vi "ManualTestingDialog.vi"(8 "error in":errorcluster) -> (0 "error out":errorcluster, 1 "检测区域":string, 2 "是否采样":bool, 3 "采样信息":T1, 4 "电压倍数":string, 5 "设置电源电压05V":string)   [LabVIEW 2014, in "Sample.lvlib"]
uses:
  Sample.lvlib
  DataBase/DataBase.lvlib
  DetectElecrodes/DetectElectros.lvlib
panel:
  out "电压范围":string
  out "电压频率":string
  out "输出电压值":string
  in  "备注":string
  in  "退出按钮":bool
  in  "开始采样":bool
  in  "电源电流":string
  in  "电源电压":string
  in  "电源频率":string="1"
  in  "采样位置":u16(ring) items=["上层膜采样", "下层膜采样"]
  in  "OK":bool
  in  "检测区域":u16(ring) items=["1区", "2区"]
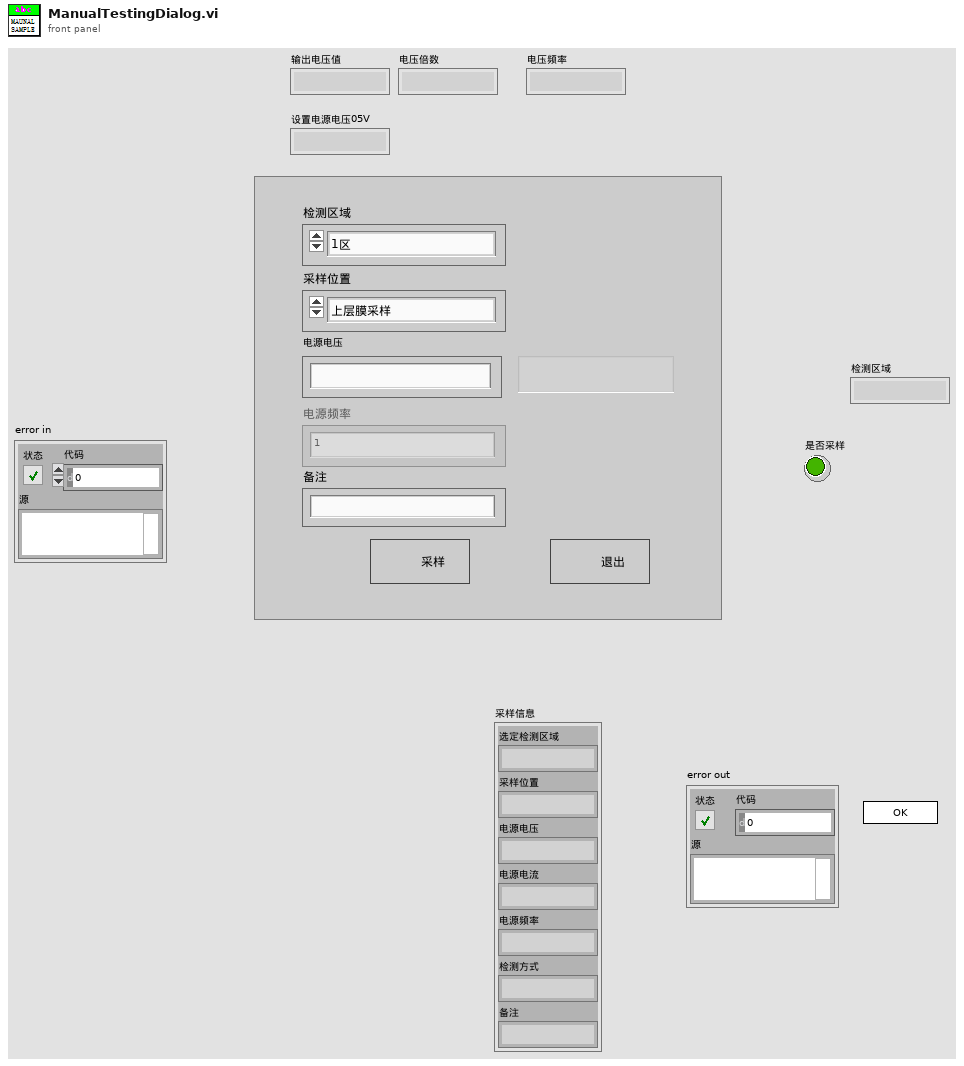
[diagram p1: front panel]
types:
  T1 = cluster{"选定检测区域":string, "采样位置":string, "电源电压":string, "电源电流":string, "电源频率":string, "检测方式":string, "备注":string}
  T2 = enum32{"invalid app kind", "Development System", "Run Time System", "Student Edition", "Embedded LabVIEW", "Evaluation", "Custom"}
  T3 = enum32{"Invalid", "Standard", "Closed", "Hidden", "Minimized", "Maximized"}
  T4 = cluster{"Core":cluster{"Current VI Reference":refnum<vi>, "Close Panel on Exit?":bool}, "Your Boolean data":bool, "Your string data":string, "采样位置":string, "检测区域":string[], "选定检测区域":cluster{"选定检测区域":string, "序号":i32}, "输出电压值":string, "电压频率":string, "电压倍数":string, "采样信息":cluster{"选定检测区域":string, "采样位置":string, "电源电压":string, "电源电流":string, "电源频率":string, "检测方式":string, "备注":string}, "最大电压":i32}
  T5 = cluster{"Current VI Reference":refnum<vi>, "Close Panel on Exit?":bool}
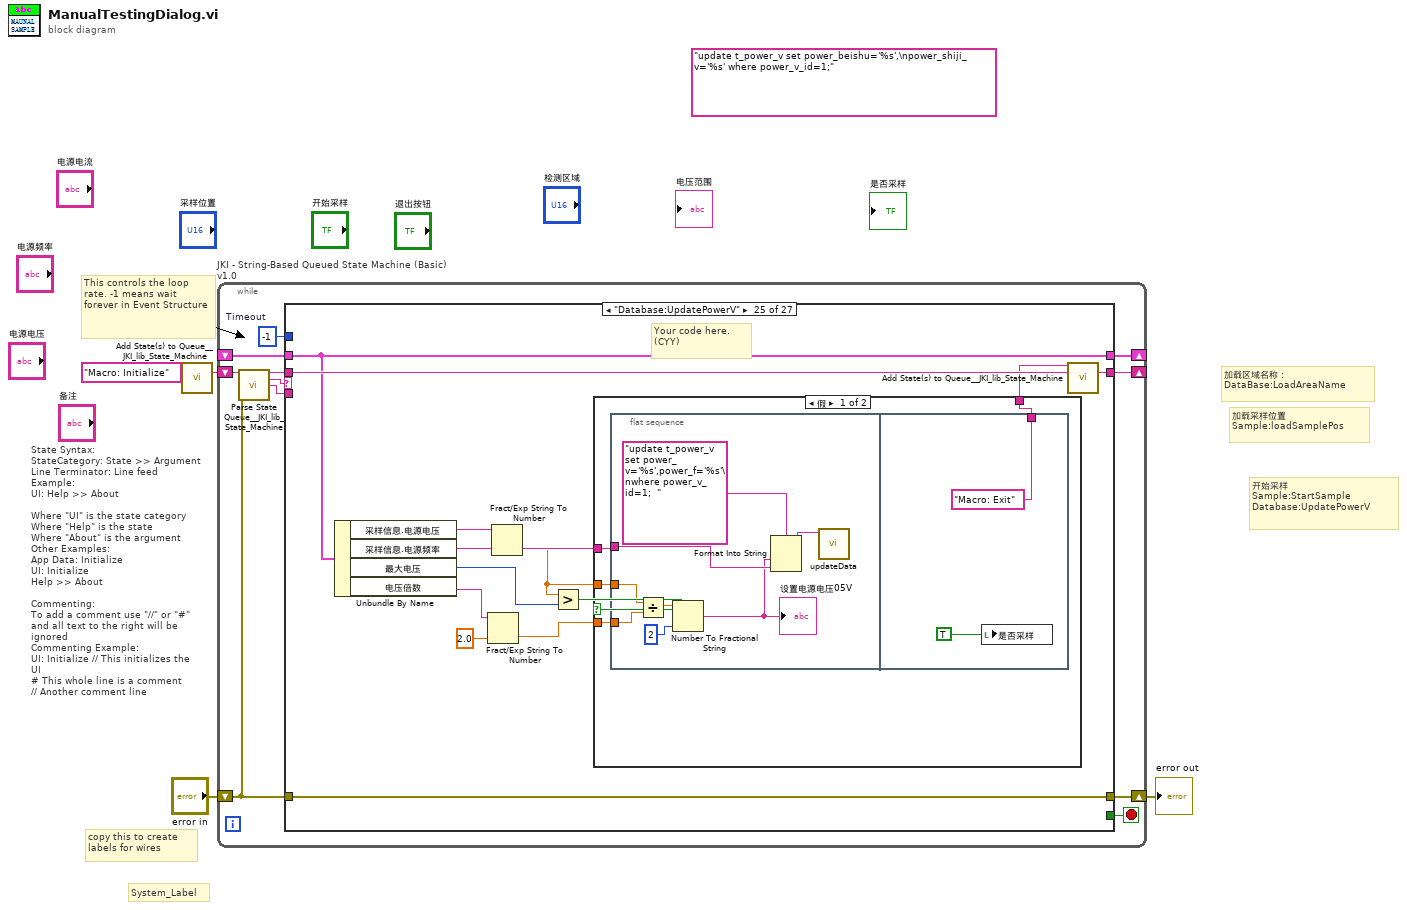
[diagram p0: block diagram]
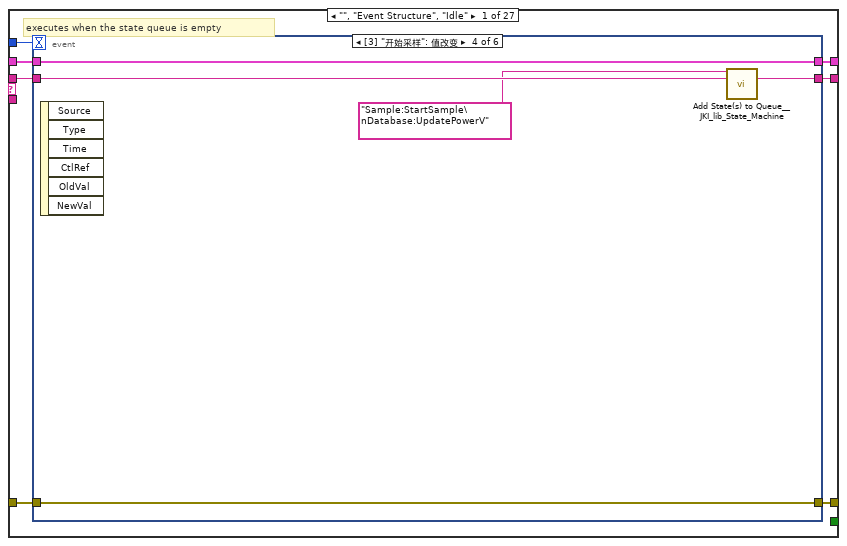
[diagram p2: hidden frame]
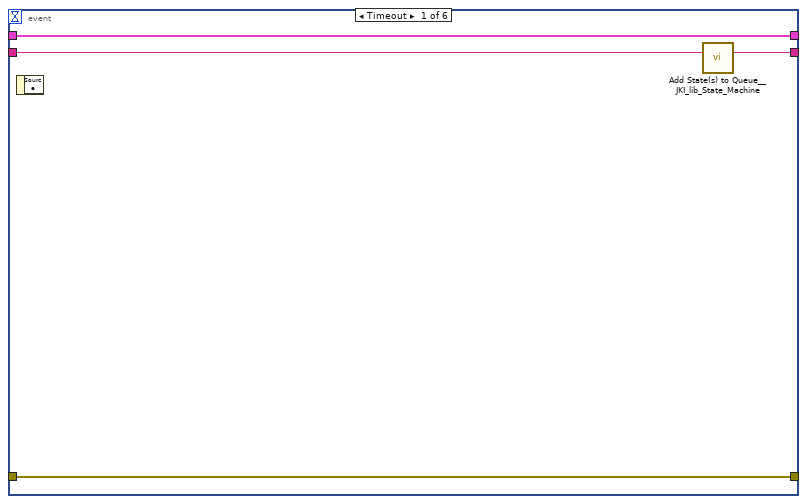
[diagram p3: hidden frame]
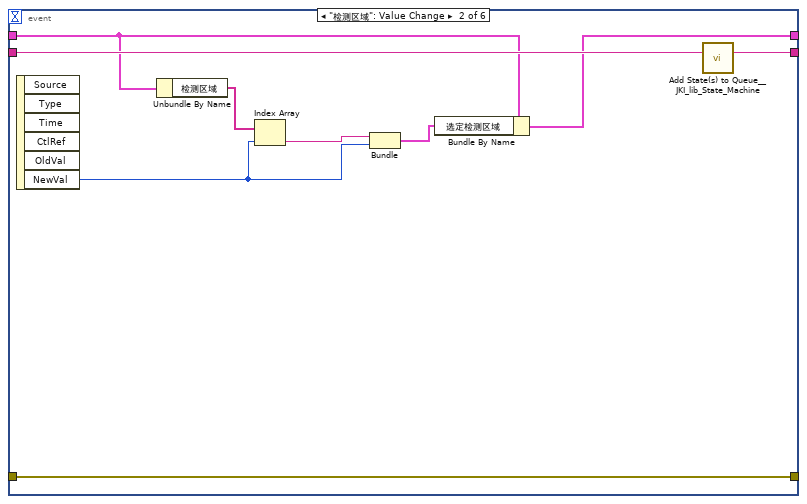
[diagram p4: hidden frame]
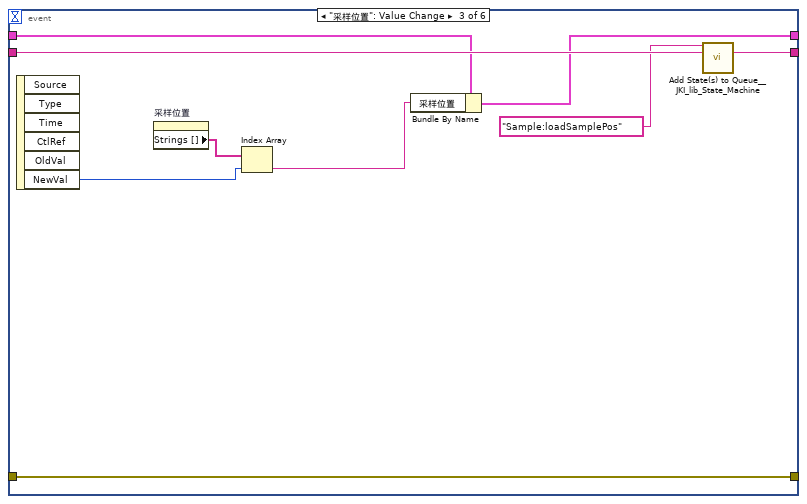
[diagram p5: hidden frame]
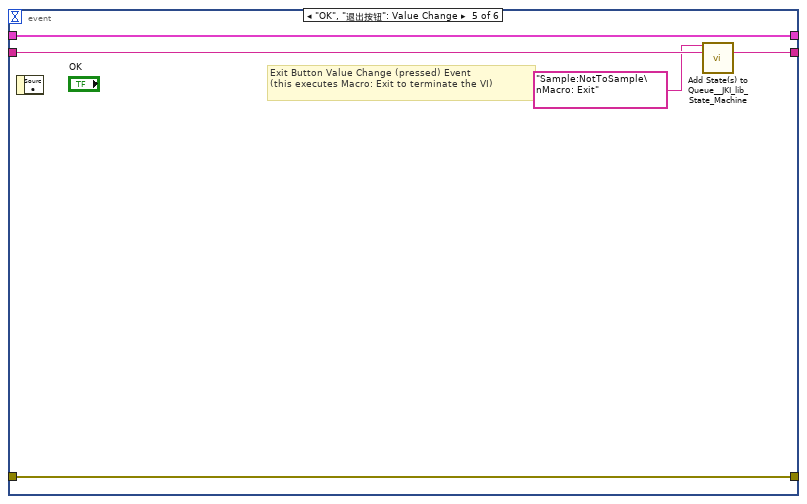
[diagram p6: hidden frame]
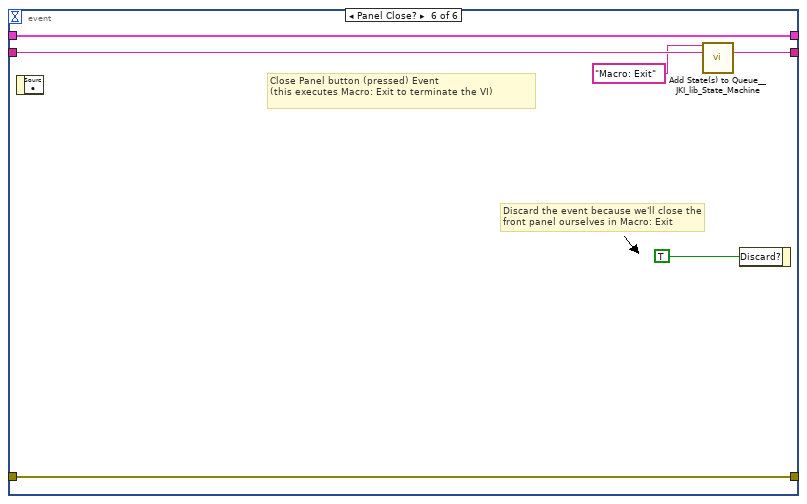
[diagram p7: hidden frame]
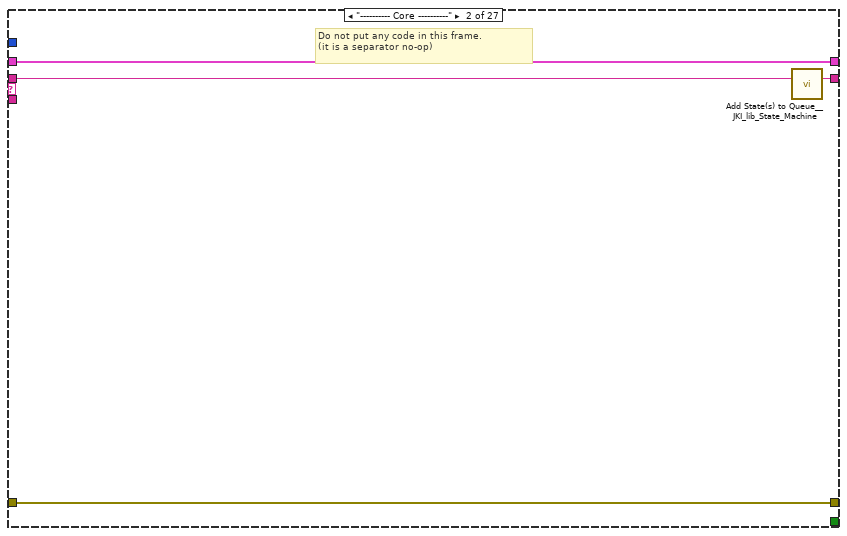
[diagram p8: hidden frame]
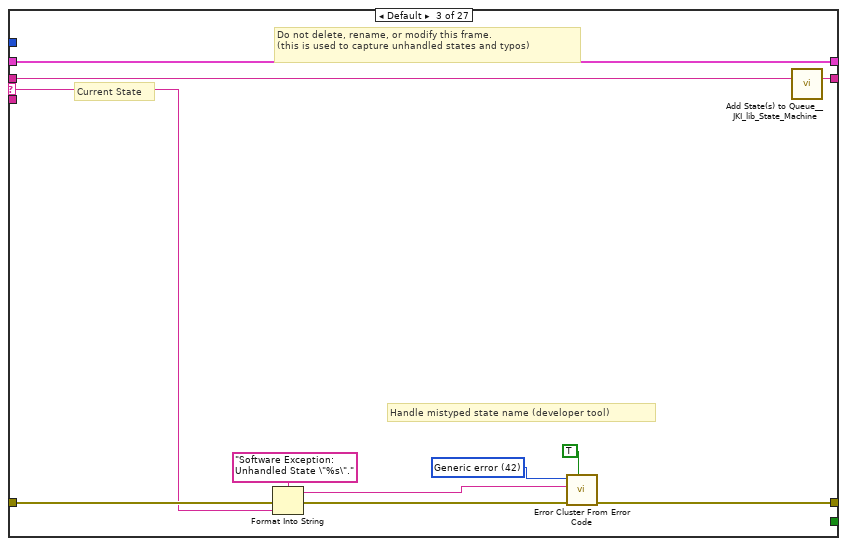
[diagram p9: hidden frame]
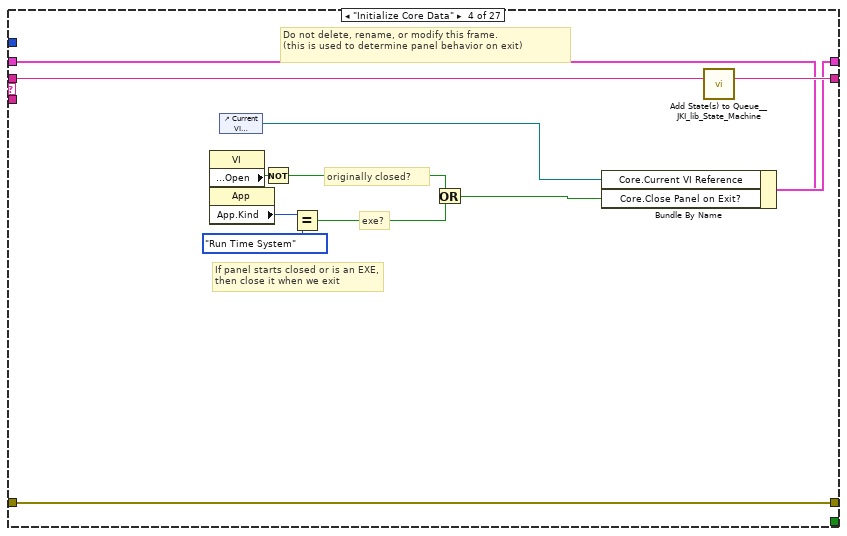
[diagram p10: hidden frame]
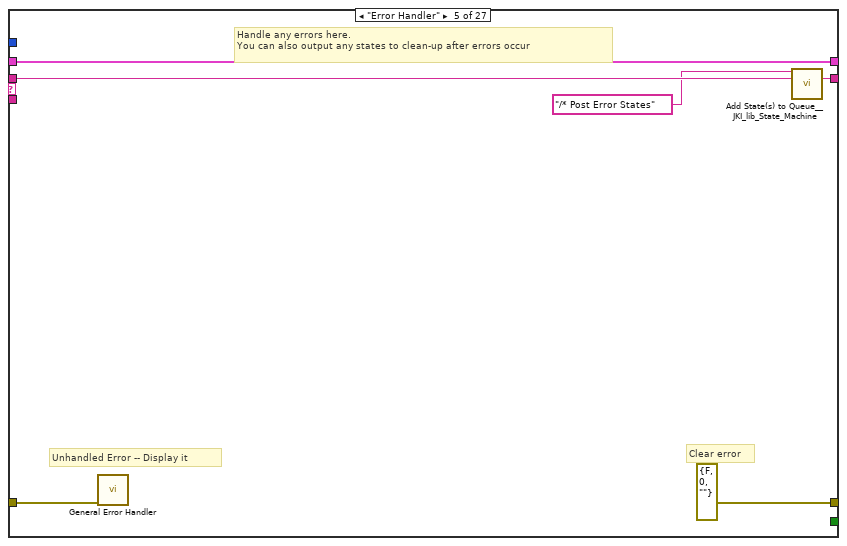
[diagram p11: hidden frame]
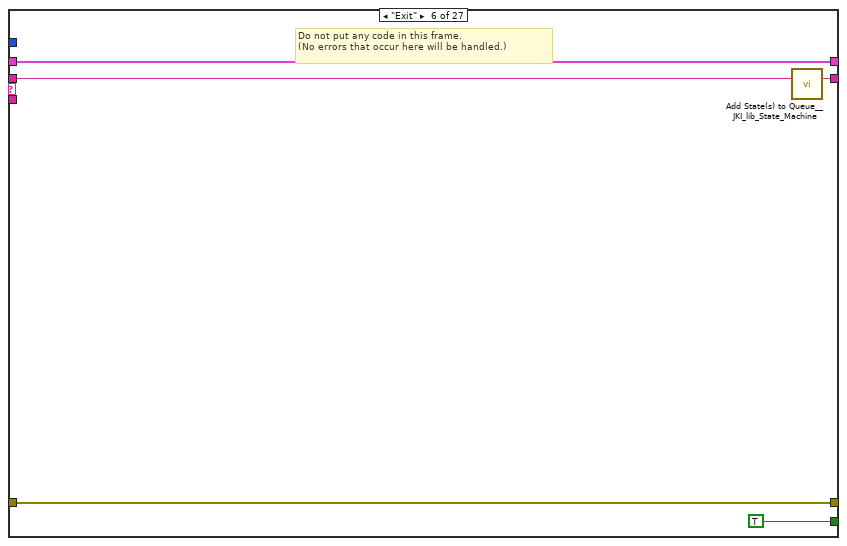
[diagram p12: hidden frame]
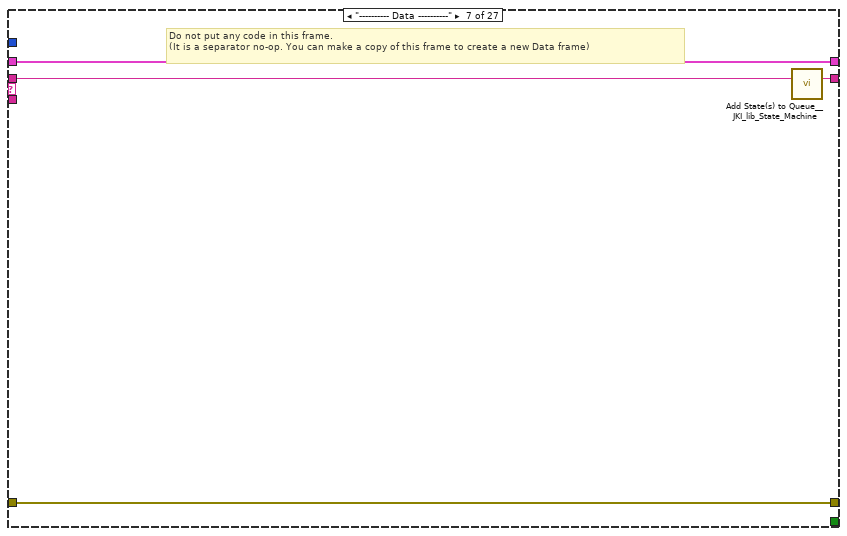
[diagram p13: hidden frame]
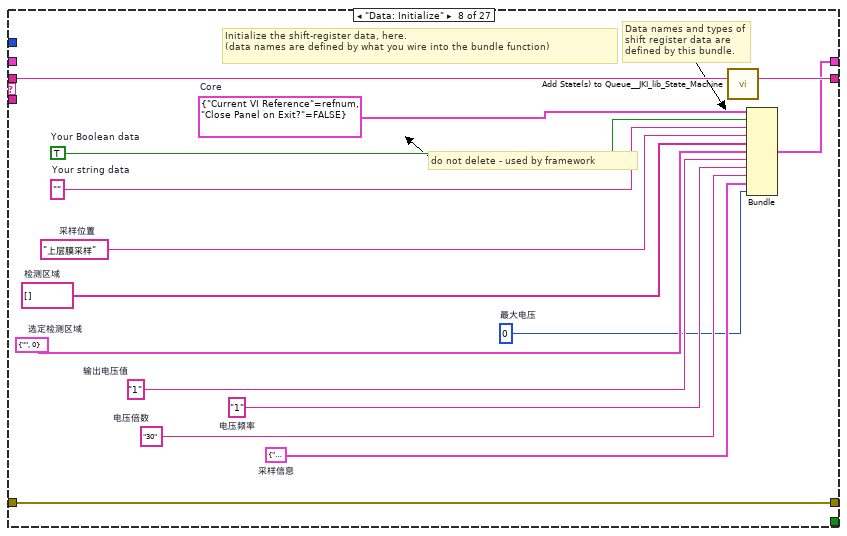
[diagram p14: hidden frame]
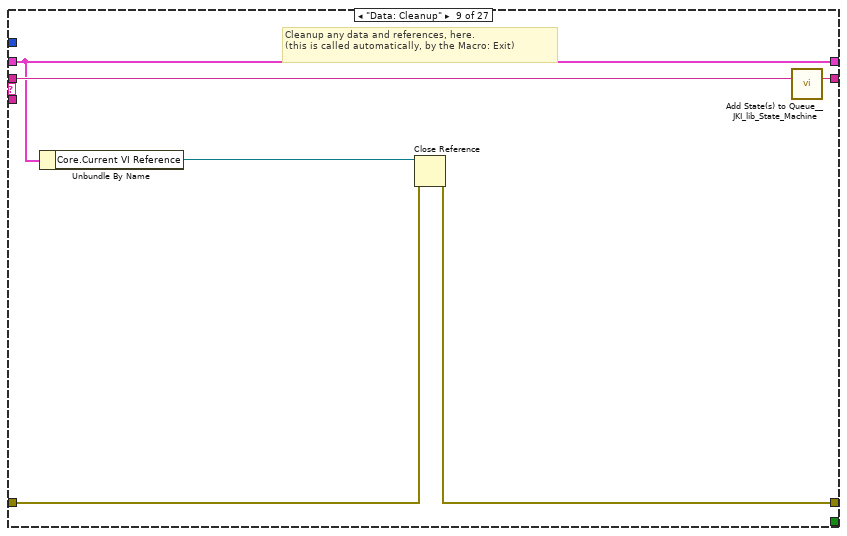
[diagram p15: hidden frame]
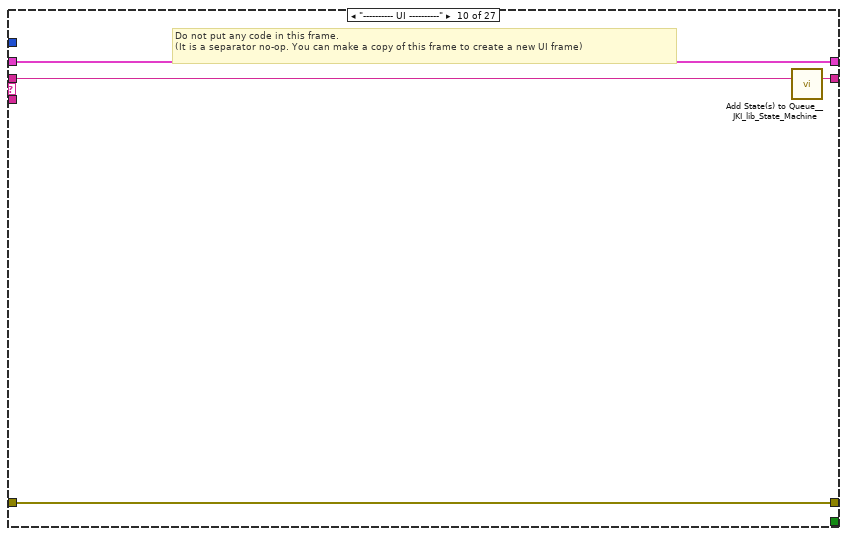
[diagram p16: hidden frame]
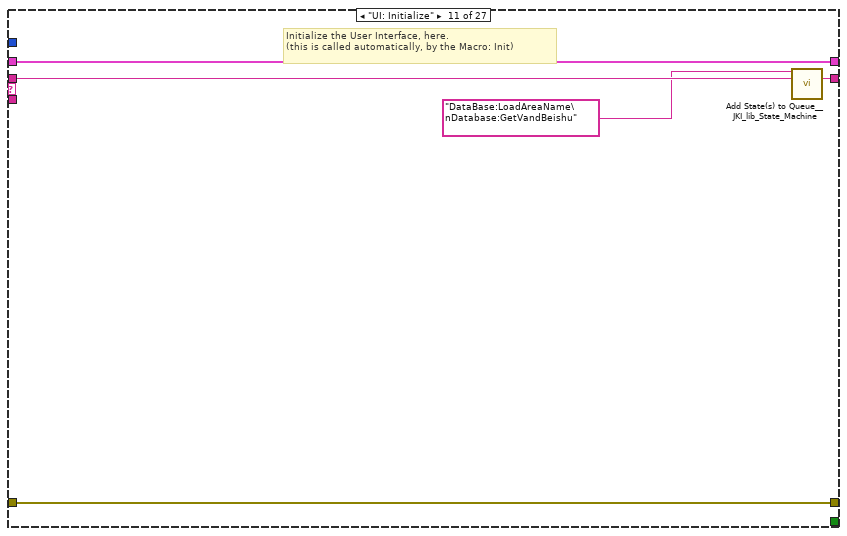
[diagram p17: hidden frame]
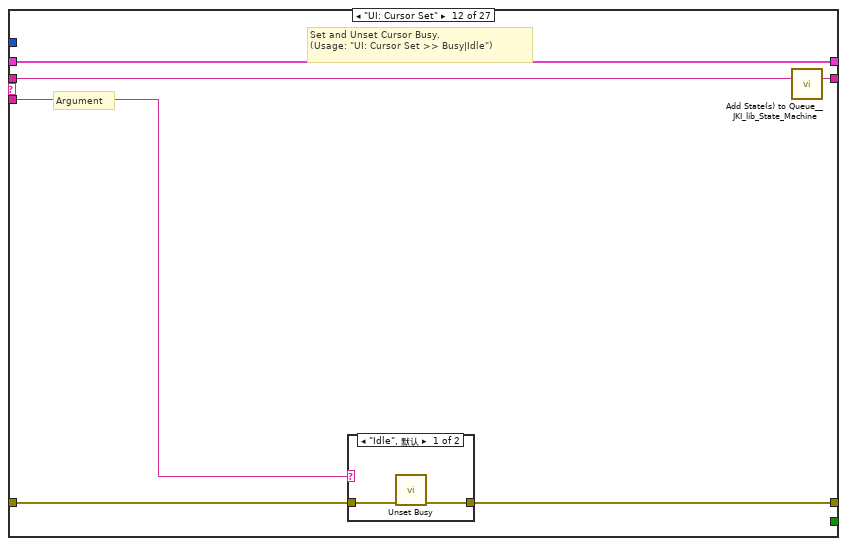
[diagram p18: hidden frame]
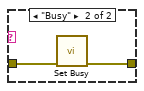
[diagram p19: hidden frame]
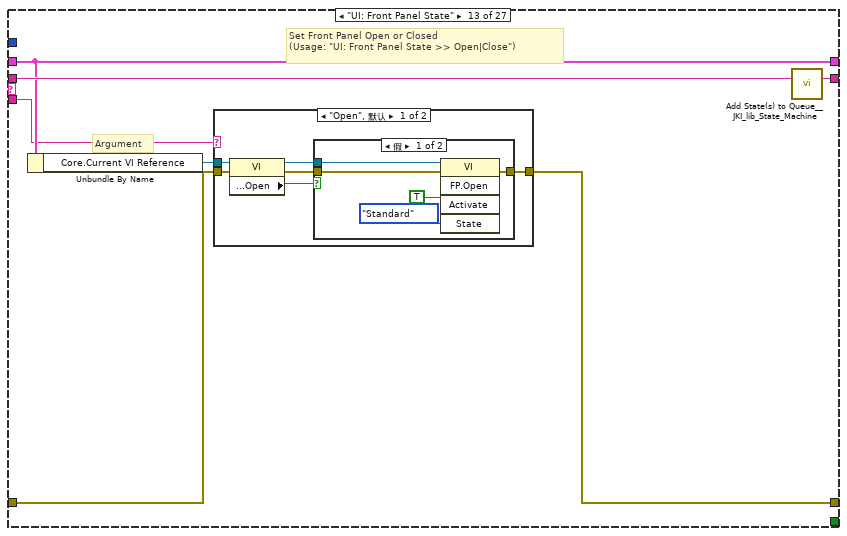
[diagram p20: hidden frame]
diagram:
  (unwired) "update t_power_v set power_beishu='%s',\npower_shiji_v='%s' where power_v_id=1;"
  # "开始采样\nSample:StartSample\nDatabase:UpdatePowerV"
  # "加载采样位置\nSample:loadSamplePos"
  # "加载区域名称：\nDataBase:LoadAreaName"
  # "State Syntax:\nStateCategory: State >> Argument\nLine Terminator: Line feed\nExample:\nUI: Help >> About\n\nWhere \"UI\" is the state category\nWhere \"Help\" is the state\nWhere \"About\" is the argument\nOther Examples:\nApp Data: Initialize\nUI: Initialize\nHelp >> About\n\nCommenting:\nTo add a comment use \"//\" or \"#\" and all text to the right will be ignored\nCommenting Example:\nUI: Initialize // This initializes the UI\n# This whole line is a comment\n// Another comment line"
  # "copy this to create labels for wires"
  # "This controls the loop rate. -1 means wait forever in Event Structure"
  # "System_Label"
  n1 = call <vilib>:"Add State(s) to Queue__JKI_lib_State_Machine.vi"("State(s) in (\"\")"="Macro: Initialize") -> ("States Out"=w4:string)  [unwired: 14 in]
  n2 = while "JKI - String-Based Queued State Machine (Basic) v1.0" {
    shift-right: [w8] -> _
    shift-left: _ -> [w7]
    shift-right: [w11] -> w2
    shift-left: "error in" -> [w5]
    shift-right: [w10] -> _
    shift-left: w4 -> [w12]
    stop <- w9 stop-if-true
    w6 = -1  # Timeout
    n3 = call <vilib>:"Parse State Queue__JKI_lib_State_Machine.vi"("State Queue"=w12, "Error In (no error)"=w5) -> ("Remaining States"=w14:string, "Current State"=w15:string, "Arguments"=w13:string)  [unwired: 11 in]
    n4 = case shown="\"Database:UpdatePowerV\"" w15 {
      selector: w15 -> [_ _ w65 _ _ _ _ _ _ _ _ _ _ _ _ _ _ _ _ _ _ _ _ _ _ _ _]
      tunnel: w14 -> [w22 w64 w69 w87 w93 w98 w102 w117 w123 w127 w132 w138 w149 w175 w180 w190 w194 w198 w202 w206 w211 w229 w233 w237 w250 w277 w291]
      tunnel: w13 -> [_ _ _ _ _ _ _ _ _ _ _ w133 w143 _ _ _ _ _ _ _ _ _ _ _ _ _ _]
      tunnel: w7 -> [w20 w61 w67 w78 w90 w96 w99 _ w118 w124 w130 w136 w145 w172 w177 w187 w191 w195 w199 w203 w208 w213 w230 w234 w247 w272 w282]
      tunnel: [w19 w62 w71 w84 errorcluster {"status"=FALSE, "code"=0, "source"=""} ("error out") w95 w100 w114 w119 w125 w129 w134 w146 w173 w178 w188 w192 w196 w200 w204 w209 w227 w231 w235 w248 w275 w289] -> w11
      tunnel: w5 -> [w18 w62 w70 w84 w89 w95 w100 w114 w120 w125 w129 w135 w147 w173 w178 w188 w192 w196 w200 w204 w209 w227 w231 w235 w248 w275 w289]
      tunnel: [w21 w63 w68 w86 w92 w97 w101 w116 w122 w126 w131 w137 w148 w174 w179 w189 w193 w197 w201 w205 w210 w228 w232 w236 w249 w276 w290] -> w10
      tunnel: [_ _ _ _ _ TRUE _ _ _ _ _ _ _ _ _ _ _ _ _ _ _ _ _ _ _ _ _] -> w9
      tunnel: [w17 w61 w67 w85 w90 w96 w99 w115 w118 w124 w130 w136 w145 w172 w177 w187 w191 w195 w199 w203 w208 w212 w230 w234 w247 w271 w281] -> w8
      tunnel: w6 -> [w16 _ _ _ _ _ _ _ _ _ _ _ _ _ _ _ _ _ _ _ _ _ _ _ _ _ _]
      frame "", "Event Structure", "Idle" {
        # "executes when the state queue is empty"
        n5 = event shown="[3] \"开始采样\": 值改变" {
          selector: _ -> [_ _ _ _ _ _]
          dyn-events: _ -> [_ _ _ _ _ _]
          timeout: w16 -> [_ _ _ _ _ _]
          tunnel: w22 -> [w26 w35 w44 w49 w54 w60]
          tunnel: [w25 w34 w43 w48 w53 w59] -> w21
          tunnel: w20 -> [w23 w31 w38 w46 w51 w57]
          tunnel: [w24 w33 w42 w47 w52 w58] -> w19
          tunnel: w18 -> [w24 w33 w42 w47 w52 w58]
          tunnel: [w23 w30 w37 w46 w51 w57] -> w17
          event Timeout {
            n6 = event-data() -> ()  [unwired: 1 in, 1 out]
            n7 = call <vilib>:"Add State(s) to Queue__JKI_lib_State_Machine.vi"("State(s) in (\"\")"=w26) -> ("States Out"=w25:string)  [unwired: 14 in]
          }
          event "检测区域": Value Change {
            n8 = event-data() -> ("NewVal"=w28:u16)  [unwired: 1 in, 5 out]
            n9 = Unbundle By Name(w31) -> ("检测区域"=w32:string[])
            n10 = Index Array(array=w32, index=w28) -> (element=w29:string)
            n11 = Bundle("data"=w29, "NewVal"=w28) -> (w27:cluster{"data":string, "NewVal":u16})  [unwired: 1 in]
            n12 = Bundle By Name(cluster=w31, "选定检测区域"=w27) -> (w30:T4)
            n13 = call <vilib>:"Add State(s) to Queue__JKI_lib_State_Machine.vi"("State(s) in (\"\")"=w35) -> ("States Out"=w34:string)  [unwired: 14 in]
          }
          event "采样位置": Value Change {
            n14 = event-data() -> ("NewVal"=w40:u16)  [unwired: 1 in, 5 out]
            n15 = property on="采样位置" class="Ring (严格)"() -> ("Strings []"=w41:string[])  [unwired: 2 in, 2 out]
            n16 = Index Array(array=w41, index=w40) -> (element=w39:string)
            n17 = Bundle By Name(cluster=w38, "采样位置"=w39) -> (w37:T4)
            n18 = call <vilib>:"Add State(s) to Queue__JKI_lib_State_Machine.vi"("State(s) in Front (\"\")"="Sample:loadSamplePos", "State(s) in (\"\")"=w44) -> ("States Out"=w43:string)  [unwired: 13 in]
          }
          event "开始采样": Value Change {
            n19 = event-data() -> ()  [unwired: 1 in, 6 out]
            n20 = call <vilib>:"Add State(s) to Queue__JKI_lib_State_Machine.vi"("State(s) in Front (\"\")"="Sample:StartSample\nDatabase:UpdatePowerV", "State(s) in (\"\")"=w49) -> ("States Out"=w48:string)  [unwired: 13 in]
          }
          event "OK", "退出按钮": Value Change {
            # "Exit Button Value Change (pressed) Event\n(this executes Macro: Exit to terminate the VI)"
            n21 = event-data() -> ()  [unwired: 1 in, 1 out]
            n22 = call <vilib>:"Add State(s) to Queue__JKI_lib_State_Machine.vi"("State(s) in Front (\"\")"="Sample:NotToSample\nMacro: Exit", "State(s) in (\"\")"=w54) -> ("States Out"=w53:string)  [unwired: 13 in]
          }
          event Panel Close? {
            # "Discard the event because we'll close the front panel ourselves in Macro: Exit"
            # "Close Panel button (pressed) Event\n(this executes Macro: Exit to terminate the VI)"
            n23 = event-data() -> ()  [unwired: 1 in, 1 out]
            n24 = call <vilib>:"Add State(s) to Queue__JKI_lib_State_Machine.vi"("State(s) in Front (\"\")"="Macro: Exit", "State(s) in (\"\")"=w60) -> ("States Out"=w59:string)  [unwired: 13 in]
            n25 = event-data("Discard?"=TRUE) -> ()  [unwired: 1 in, 1 out]
          }
        }
      }
      frame "---------- Core ----------" {
        # "Do not put any code in this frame.\n(it is a separator no-op)"
        n26 = call <vilib>:"Add State(s) to Queue__JKI_lib_State_Machine.vi"("State(s) in (\"\")"=w64) -> ("States Out"=w63:string)  [unwired: 14 in]
      }
      frame Default {
        w74 = 42 items=["No error", "Argument error", "Memory is full", "Out of zone", "End of file", "File already open", "Generic file I/O error", "File not found", "File permission error", "Disk is full", "Duplicate path", "Too many files open", "System feature not enabled", "Resource file not found", "Cannot add resource", "Resource not found", "Image not found", "Image memory error", "Pen does not exist", "Config type invalid", "Config token not found", "Config parse error", "Config memory error", "Bad external code format", "Bad external code offset", "External code not present", "Null window", "Destroy window error", "Null menu", "Print aborted", "Bad print record", "Print driver error", "Windows error during printing", "Memory error during printing", "Print dialog error", "Generic print error", "Invalid device refnum", "Device not found", "Device parameter error", "Device unit error", "Cannot open device", "Device call aborted", "Generic error", "Cancelled by user", "Object ID too low", "Object ID too high", "Object not in heap", "Unknown heap", "Unknown object (invalid DefProc)", "Unknown object (DefProc not in table)", "Message out of range", "Invalid (null) method", "Unknown message", "Manager call not supported", "Bad address", "Network operation in progress", "Network operation timed out", "Connection is busy", "Network attribute not supported", "Network error", "Address in use", "System out of memory", "Connection aborted", "Connection refused", "Not connected", "Already connected", "Connection closed", "Initialization error (interapplication manager)", "Bad occurrence", "Wait on unbound occurrence handler", "Occurrence queue overflow", "Datalog type conflict", "Unused", "Unrecognized type (interapplication manager)", "Memory corrupt", "Failed to make temporary DLL", "Old CIN version", "Drag socket not found", "Failed to load drop-object", "Failed to register OLE object", "Failed to release OLE object", "Format specifier type mismatch", "Unknown format specifier", "Too few format specifiers", "Too many format specifiers", "Scan failed", "Newer CIN version", "Error converting to variant", "Runtime menu error", "Password tampered", "Variant attribute not found", "Incompatible variant data type", "Event data is not available", "Event Store is not present", "Occurrence is not found", "Event Queue is not created", "Event info is not available", "Refnum passed is NULL", "Error retrieving Class GUID", "Error retrieving CoClass GUID", "Error retrieving TypeLib GUID.", "Bad built application magic bytes.", "Specific driver is different from the specific driver associated with the Logical Name.", "There is no session opened to the class driver.", "Max Error", "MAX - Error with config objects", "MAX - Error loading configuration", "MAX - Group not supported"]
        # "Current State"
        # "Do not delete, rename, or modify this frame.\n(this is used to capture unhandled states and typos)"
        # "Handle mistyped state name (developer tool)"
        n27 = Format Into String(format string="Software Exception: Unhandled State \"%s\"." ("message"), error in=w70, w65) -> (resulting string=w73:string, error out=w72:errorcluster)  [unwired: 1 in]
        n28 = call <vilib>:"Error Cluster From Error Code.vi"("show call chain? (False)"=TRUE, "error in (no error)"=w72, "error message (\"\")"=w73, "error code (0)"=w74) -> ("error out"=w71:errorcluster)  [unwired: 5 in]
        n29 = call <vilib>:"Add State(s) to Queue__JKI_lib_State_Machine.vi"("State(s) in (\"\")"=w69) -> ("States Out"=w68:string)  [unwired: 14 in]
      }
      frame "Initialize Core Data" {
        # "Do not delete, rename, or modify this frame.\n(this is used to determine panel behavior on exit)"
        # "originally closed?"
        # "exe?"
        # "If panel starts closed or is an EXE, then close it when we exit"
        n30 = property class="VI"() -> ("Front Panel.Open"=w83:bool)  [unwired: 2 in, 2 out]
        n31 = property class="App"() -> ("App.Kind"=w82:T2)  [unwired: 2 in, 2 out]
        n32 = control-ref of="Current VI Reference"() -> (w76:refnum<vi>)
        n33 = Not(x=w83) -> (.not. x?=w80:bool)
        n34 = Equal?(x=w82, y=T2."Run Time System" ("Application:Kind")) -> (x = y?=w79:bool)
        n35 = Or(x=w80, y=w79) -> (x .or. y?=w77:bool)
        n36 = Bundle By Name(cluster=w78, "Core.Current VI Reference"=w76, "Core.Close Panel on Exit?"=w77) -> (w85:T4)
        n37 = call <vilib>:"Add State(s) to Queue__JKI_lib_State_Machine.vi"("State(s) in (\"\")"=w87) -> ("States Out"=w86:string)  [unwired: 14 in]
      }
      frame "Error Handler" {
        # "Unhandled Error -- Display it"
        # "Handle any errors here.\nYou can also output any states to clean-up after errors occur"
        # "Clear error"
        n38 = call <vilib>:"General Error Handler.vi"("error in (no error)"=w89) -> ()  [unwired: 10 in, 5 out]
        n39 = call <vilib>:"Add State(s) to Queue__JKI_lib_State_Machine.vi"("State(s) in Front (\"\")"="/* Post Error States", "State(s) in (\"\")"=w93) -> ("States Out"=w92:string)  [unwired: 13 in]
      }
      frame "Exit" {
        # "Do not put any code in this frame.\n(No errors that occur here will be handled.)"
        n40 = call <vilib>:"Add State(s) to Queue__JKI_lib_State_Machine.vi"("State(s) in (\"\")"=w98) -> ("States Out"=w97:string)  [unwired: 14 in]
      }
      frame "---------- Data ----------" {
        # "Do not put any code in this frame.\n(It is a separator no-op. You can make a copy of this frame to create a new Data frame)"
        n41 = call <vilib>:"Add State(s) to Queue__JKI_lib_State_Machine.vi"("State(s) in (\"\")"=w102) -> ("States Out"=w101:string)  [unwired: 14 in]
      }
      frame "Data: Initialize" {
        w103 = 0  # 最大电压
        w104 = T1 {"选定检测区域"="", "采样位置"="", "电源电压"="", "电源电流"="", "电源频率"="", "检测方式"="", "备注"=""}  # 采样信息
        w105 = "30"  # 电压倍数
        w106 = "1"  # 电压频率
        w107 = "1"  # 输出电压值
        w108 = cluster{"选定检测区域":string, "序号":i32} {"选定检测区域"="", "序号"=0}  # 选定检测区域
        w109 = string[] []  # 检测区域
        w110 = "上层膜采样"  # 采样位置
        w111 = T5 {"Current VI Reference"=refnum, "Close Panel on Exit?"=FALSE}  # Core
        w113 = TRUE  # Your Boolean data
        w112 = ""  # Your string data
        # "do not delete - used by framework"
        # "Data names and types of shift register data are defined by this bundle."
        # "Initialize the shift-register data, here.\n(data names are defined by what you wire into the bundle function)"
        n42 = call <vilib>:"Add State(s) to Queue__JKI_lib_State_Machine.vi"("State(s) in (\"\")"=w117) -> ("States Out"=w116:string)  [unwired: 14 in]
        n43 = Bundle("Core"=w111, "Your Boolean data"=w113, "Your string data"=w112, "采样位置"=w110, "检测区域"=w109, "选定检测区域"=w108, "输出电压值"=w107, "电压频率"=w106, "电压倍数"=w105, "采样信息"=w104, "最大电压"=w103) -> (w115:T4)  [unwired: 1 in]
      }
      frame "Data: Cleanup" {
        # "Cleanup any data and references, here.\n(this is called automatically, by the Macro: Exit)"
        n44 = Unbundle By Name(w118) -> ("Core.Current VI Reference"=w121:refnum<vi>)
        n45 = Close Reference(reference=w121, error in (no error)=w120) -> (error out=w119:errorcluster)
        n46 = call <vilib>:"Add State(s) to Queue__JKI_lib_State_Machine.vi"("State(s) in (\"\")"=w123) -> ("States Out"=w122:string)  [unwired: 14 in]
      }
      frame "---------- UI ----------" {
        # "Do not put any code in this frame.\n(It is a separator no-op. You can make a copy of this frame to create a new UI frame)"
        n47 = call <vilib>:"Add State(s) to Queue__JKI_lib_State_Machine.vi"("State(s) in (\"\")"=w127) -> ("States Out"=w126:string)  [unwired: 14 in]
      }
      frame "UI: Initialize" {
        # "Initialize the User Interface, here.\n(this is called automatically, by the Macro: Init)"
        n48 = call <vilib>:"Add State(s) to Queue__JKI_lib_State_Machine.vi"("State(s) in Front (\"\")"="DataBase:LoadAreaName\nDatabase:GetVandBeishu", "State(s) in (\"\")"=w132) -> ("States Out"=w131:string)  [unwired: 13 in]
      }
      frame "UI: Cursor Set" {
        # "Argument"
        # "Set and Unset Cursor Busy.\n(Usage: \"UI: Cursor Set >> Busy|Idle\")"
        n49 = case shown="\"Idle\", 默认" w133 {
          tunnel: w135 -> [w140 w142]
          tunnel: [w139 w141] -> w134
          frame "Idle", Default {
            n50 = call <vilib>:"Unset Busy.vi"("error in (no error)"=w140) -> ("error out"=w139:errorcluster)  [unwired: 10 in]
          }
          frame "Busy" {
            n51 = call <vilib>:"Set Busy.vi"("error in (no error)"=w142) -> ("error out"=w141:errorcluster)  [unwired: 9 in, 1 out]
          }
        }
        n52 = call <vilib>:"Add State(s) to Queue__JKI_lib_State_Machine.vi"("State(s) in (\"\")"=w138) -> ("States Out"=w137:string)  [unwired: 14 in]
      }
      frame "UI: Front Panel State" {
        # "Argument"
        # "Set Front Panel Open or Closed\n(Usage: \"UI: Front Panel State >> Open|Close\")"
        n53 = Unbundle By Name(w145) -> ("Core.Current VI Reference"=w144:refnum<vi>)
        n54 = case shown="\"Open\", 默认" w143 {
          tunnel: w147 -> [w153 w166]
          tunnel: [w155 w167] -> w146
          tunnel: w144 -> [w154 w164]
          frame "Open", Default {
            n55 = property class="VI"(reference=w154, error in=w153) -> (reference out=w151:refnum<vi>, error out=w152:errorcluster, "Front Panel.Open"=w150:bool)
            n56 = case shown="假" w150 {
              tunnel: [w158 w161] -> w155
              tunnel: w152 -> [w157 w161]
              tunnel: w151 -> [w156 _]
              frame False {
                n57 = invoke class="VI" method="FP.Open"(reference=w156, error in=w157, "Activate"=TRUE, "State"=T3."Standard") -> (error out=w158:errorcluster)  [unwired: 1 in, 4 out]
              }
              frame True {
              }
            }
          }
          frame "Close" {
            n58 = property class="VI"(reference=w164, error in=w166) -> (reference out=w163:refnum<vi>, error out=w165:errorcluster, "Front Panel.Open"=w162:bool)
            n59 = case shown="真" w162 {
              tunnel: [w168 w171] -> w167
              tunnel: w165 -> [w168 w170]
              tunnel: w163 -> [_ w169]
              frame False {
              }
              frame True {
                n60 = invoke class="VI" method="FP.Close"(reference=w169, error in=w170) -> (error out=w171:errorcluster)  [unwired: 1 in, 2 out]
              }
            }
          }
        }
        n61 = call <vilib>:"Add State(s) to Queue__JKI_lib_State_Machine.vi"("State(s) in (\"\")"=w149) -> ("States Out"=w148:string)  [unwired: 14 in]
      }
      frame "---------- Macro ----------" {
        # "Do not put any code in this frame.\n(It is a separator no-op. You can make a copy of this frame to create a new Macro frame)"
        n62 = call <vilib>:"Add State(s) to Queue__JKI_lib_State_Machine.vi"("State(s) in (\"\")"=w175) -> ("States Out"=w174:string)  [unwired: 14 in]
      }
      frame "Macro: Initialize" {
        w176 = "Data: Initialize\nInitialize Core Data\nUI: Initialize\nUI: Front Panel State >> Open"  # Data: Initialize Initialize Core Data UI: Initialize UI: Front Panel State >> Open
        # "Initialization Macro\n(This is called once, when the VI starts)"
        n63 = call <vilib>:"Add State(s) to Queue__JKI_lib_State_Machine.vi"("State(s) in Front (\"\")"=w176, "State(s) in (\"\")"=w180) -> ("States Out"=w179:string)  [unwired: 13 in]
      }
      frame "Macro: Exit" {
        # "Exit Macro\n(This is called once, when the VI exits)"
        n64 = Unbundle By Name(w187) -> ("Core.Close Panel on Exit?"=w186:bool)
        n65 = Select(t="UI: Front Panel State >> Close", s=w186, f="") -> (s? t:f=w183:string)
        n66 = call <vilib>:"Add State(s) to Queue__JKI_lib_State_Machine.vi"("State(s) in (\"\")"=w183, "State(s) at Back (\"\")"="Data: Cleanup\nExit") -> ("States Out"=w181:string)  [unwired: 13 in]
        n67 = call <vilib>:"Add State(s) to Queue__JKI_lib_State_Machine.vi"("State(s) in Front (\"\")"=w181, "State(s) in (\"\")"=w190) -> ("States Out"=w189:string)  [unwired: 13 in]
      }
      frame "---------- New Category ----------" {
        # "Template Separator\n(You can make a copy of, or modify, this frame)"
        n68 = call <vilib>:"Add State(s) to Queue__JKI_lib_State_Machine.vi"("State(s) in (\"\")"=w194) -> ("States Out"=w193:string)  [unwired: 14 in]
      }
      frame "New Category: 1" {
        # "Your code here.\n(You can make a copy of, or modify, this frame)"
        n69 = call <vilib>:"Add State(s) to Queue__JKI_lib_State_Machine.vi"("State(s) in (\"\")"=w198) -> ("States Out"=w197:string)  [unwired: 14 in]
      }
      frame "New Category: 2" {
        # "Your code here.\n(You can make a copy of, or modify, this frame)"
        n70 = call <vilib>:"Add State(s) to Queue__JKI_lib_State_Machine.vi"("State(s) in (\"\")"=w202) -> ("States Out"=w201:string)  [unwired: 14 in]
      }
      frame "-------------Sample----------" {
        # "Your code here.\n(You can make a copy of, or modify, this frame)"
        n71 = call <vilib>:"Add State(s) to Queue__JKI_lib_State_Machine.vi"("State(s) in (\"\")"=w206) -> ("States Out"=w205:string)  [unwired: 14 in]
      }
      frame "Sample:NotToSample" {
        n72 = local write "是否采样"(FALSE) -> ()
        n73 = call <vilib>:"Add State(s) to Queue__JKI_lib_State_Machine.vi"("State(s) in (\"\")"=w211) -> ("States Out"=w210:string)  [unwired: 14 in]
      }
      frame "Sample:StartSample" {
        # "在这设置：采样信息\n1、保存到t_power_v表中\n2、判断是否超过电压值\n3、"
        # "Your code here.\n(You can make a copy of, or modify, this frame)"
        n74 = local read "采样位置"() -> (w219:u16)
        n75 = local read "检测区域"() -> (w221:u16)
        n76 = local read "备注"() -> (w216:string)
        n77 = local read "电源电压"() -> (w215:string)
        n78 = local read "电源电流"() -> (w224:string)
        n79 = local read "电源频率"() -> (w223:string)
        n80 = Unbundle By Name(w213) -> ("检测区域"=w226:string[])
        n81 = property on="采样位置" class="Ring (严格)"() -> ("Strings []"=w220:string[])  [unwired: 2 in, 2 out]
        n82 = Index Array(array=w220, index=w219) -> (element=w218:string)
        n83 = Index Array(array=w226, index=w221) -> (element=w225:string)
        n84 = Bundle By Name(cluster=T1 {"选定检测区域"="", "采样位置"="", "电源电压"="", "电源电流"="", "电源频率"="", "检测方式"="", "备注"=""} ("输入簇"), "选定检测区域"=w225, "采样位置"=w218, "电源电压"=w215, "电源电流"=w224, "电源频率"=w223, "检测方式"="手动检测", "备注"=w216) -> (w214:T1)
        "采样信息" <- w214
        n85 = Bundle By Name(cluster=w213, "采样信息"=w214) -> (w212:T4)
        n86 = call <vilib>:"Add State(s) to Queue__JKI_lib_State_Machine.vi"("State(s) in (\"\")"=w229) -> ("States Out"=w228:string)  [unwired: 14 in]
      }
      frame "Sample:loadSamplePos" {
        # "Your code here.\n(You can make a copy of, or modify, this frame)"
        n87 = call <vilib>:"Add State(s) to Queue__JKI_lib_State_Machine.vi"("State(s) in (\"\")"=w233) -> ("States Out"=w232:string)  [unwired: 14 in]
      }
      frame "-----------DataBase------------" {
        # "Your code here.\n(You can make a copy of, or modify, this frame)"
        n88 = call <vilib>:"Add State(s) to Queue__JKI_lib_State_Machine.vi"("State(s) in (\"\")"=w237) -> ("States Out"=w236:string)  [unwired: 14 in]
      }
      frame "Database:UpdatePowerV" {
        # "Your code here.\n(CYY)"
        n89 = Unbundle By Name(w247) -> ("采样信息.电源电压"=w243:string, "采样信息.电源频率"=w244:string, "最大电压"=w246:i32, "电压倍数"=w241:string)
        n90 = Fract/Exp String To Number(string=w241, default (0 dbl)=2.0 ("默认(0 DBL)")) -> (number=w240:dbl)  [unwired: 2 in, 1 out]
        n91 = Fract/Exp String To Number(string=w243) -> (number=w242:dbl)  [unwired: 3 in, 1 out]
        n92 = Greater?(x=w242, y=w246) -> (0:w245:bool)
        n93 = case shown="假" w245 {
          tunnel: w244 -> [w254 _]
          tunnel: w240 -> [w253 _]
          tunnel: w242 -> [w252 _]
          tunnel: [w251 ""] -> w238
          frame False {
            n94 = flat-sequence {
              tunnel: w254 -> [w260]
              tunnel: w253 -> [w259]
              tunnel: w252 -> [w258]
              tunnel: ["Macro: Exit"] -> w251
              frame #0 {
                n95 = Divide(x=w258, y=w259) -> (x/y=w257:dbl)
                n96 = Number To Fractional String(number=w257, precision (6)=i16 2 ("精度(6)")) -> (F-format string=w256:string)  [unwired: 2 in]
                "设置电源电压05V" <- w256
                n97 = Format Into String(format string="update t_power_v set power_v='%s',power_f='%s'\nwhere power_v_id=1;  ", w256, w260) -> (resulting string=w262:string)  [unwired: 2 in, 1 out]
                n98 = call "updateData.vi"("SQL query"=w262) -> ()  [unwired: 10 in, 1 out]
              }
              frame #1 {
                n99 = local write "是否采样"(TRUE) -> ()
              }
            }
          }
          frame True {
            n100 = local write "是否采样"(FALSE) -> ()
            n101 = One Button Dialog(message="输入电压超过限制，请从新输入" ("消息")) -> ()  [unwired: 1 in, 1 out]
          }
        }
        n102 = call <vilib>:"Add State(s) to Queue__JKI_lib_State_Machine.vi"("State(s) in Front (\"\")"=w238, "State(s) in (\"\")"=w250) -> ("States Out"=w249:string)  [unwired: 13 in]
      }
      frame "Database:GetVandBeishu" {
        # "Your code here.\n(You can make a copy of, or modify, this frame)"
        n103 = call "GetVandBeishu.vi"() -> ("电压倍数"=w270:string, "电压频率"=w274:string, "输出电压值"=w273:string)  [unwired: 9 in]
        "输出电压值" <- w273
        "电压频率" <- w274
        "电压倍数" <- w270
        n104 = call "ZhuanVbeishu.vi"("电压倍数"=w270) -> ("电压范围"=w269:string, "最大电压值"=w268:i32)  [unwired: 9 in]
        n105 = Bundle By Name(cluster=w272, "输出电压值"=w273, "电压频率"=w274, "电压倍数"=w270, "最大电压"=w268) -> (w271:T4)
        n106 = property on="电压范围" class="Str"("Text.Text"=w269) -> ()  [unwired: 2 in, 2 out]
        n107 = call <vilib>:"Add State(s) to Queue__JKI_lib_State_Machine.vi"("State(s) in (\"\")"=w277) -> ("States Out"=w276:string)  [unwired: 14 in]
      }
      frame "DataBase:LoadAreaName" {
        # "Your code here.\n(You can make a copy of, or modify, this frame)"
        n108 = call "SelectData.vi"("SQL query"="select area_name from t_area") -> ("recordset data"=w285:variant[][])  [unwired: 7 in, 1 out]
        n109 = call "ReadDataFromDatabase.vi"("长度"=1, "index"=0, "recordset data"=w285) -> ("所有记录"=w284:string[][])  [unwired: 7 in, 1 out]
        n110 = Index Array(array=w284, index (col)=0) -> (element=w280:string[])  [unwired: 1 in]
        n111 = local read "检测区域"() -> (w279:u16)
        n112 = Bundle By Name(cluster=w282, "检测区域"=w280) -> (w281:T4)
        n113 = property on="检测区域" class="Ring (严格)"("Strings []"=w280) -> ()  [unwired: 2 in, 2 out]
        n114 = Index Array(array=w280, index=w279) -> (element=→"检测区域":string)
        n115 = call <vilib>:"Add State(s) to Queue__JKI_lib_State_Machine.vi"("State(s) in (\"\")"=w291) -> ("States Out"=w290:string)  [unwired: 14 in]
      }
    }
  }
  "error out" <- w2
